vi "nanocal -- nuclear schottky fit V4.vi"() -> ()   [LabVIEW 2020] (continued)
\"mm2\"-> 0.000000000000  , \"mm3\"-> 0.000000000000  , \"T\"->  1.130000000000  , \"B\"-> 12.000000000000  , \"θ\"-> 60.000000000000  |>   , \r\"IDS0371_210908_RAW_cal__ref_\" ->   <| \"ζ\"->  0.020664849580  , \"τ1\"-> 0.018108723176  , \"τS\"-> 0.010299896170  , \"τN\"-> 0.000079818017  , \"τC\"-> 0.006259144045  , \"κ0\"-> 0.000000013130  , \"mm1\"-> 0.000000000000  , \"mm2\"-> 0.000000000000  , \"mm3\"-> 0.000000000000  , \"T\"->  1.900000000000  , \"B\"-> 12.000000000000  , \"θ\"-> 60.000000000000  |>   , \r\"IDS0371_210908_RAW_cal__sam_\" ->   <| \"ζ\"->  0.000000000000  , \"τ1\"-> 0.000000000000  , \"τS\"-> 0.000000000000  , \"τN\"-> 0.000000000000  , \"τC\"-> 0.000000000000  , \"κ0\"-> 0.000000000000  , \"mm1\"-> 0.000000000000  , \"mm2\"-> 0.000000000000  , \"mm3\"-> 0.000000000000  , \"T\"->  1.900000000000  , \"B\"-> 12.000000000000  , \"θ\"-> 60.000000000000  |>   , \r\"IDS0372_210908_RAW_cal__ref_\" ->   <| \"ζ\"->  0.021592146431  , \"τ1\"-> 0.018093446545  , \"τS\"-> 0.007071841556  , \"τN\"-> 0.000029085223  , \"τC\"-> 0.005341206531  , \"κ0\"-> 0.000000023517  , \"mm1\"-> 0.000000000000  , \"mm2\"-> 0.000000000000  , \"mm3\"-> 0.000000000000  , \"T\"->  3.110000000000  , \"B\"-> 12.000000000000  , \"θ\"-> 60.000000000000  |>   , \r\"IDS0372_210908_RAW_cal__sam_\" ->   <| \"ζ\"->  0.000000000000  , \"τ1\"-> 0.000000000000  , \"τS\"-> 0.000000000000  , \"τN\"-> 0.000000000000  , \"τC\"-> 0.000000000000  , \"κ0\"-> 0.000000000000  , \"mm1\"-> 0.000000000000  , \"mm2\"-> 0.000000000000  , \"mm3\"-> 0.000000000000  , \"T\"->  3.110000000000  , \"B\"-> 12.000000000000  , \"θ\"-> 60.000000000000  |>   , \r\"IDS0373_210908_RAW_cal__ref_\" ->   <| \"ζ\"->  0.028148688120  , \"τ1\"-> 0.012706961955  , \"τS\"-> 0.003881518121  , \"τN\"-> 0.000007160132  , \"τC\"-> 0.004346615253  , \"κ0\"-> 0.000000058313  , \"mm1\"-> 0.000000000000  , \"mm2\"-> 0.000000000000  , \"mm3\"-> 0.000000000000  , \"T\"->  5.750000000000  , \"B\"-> 12.000000000000  , \"θ\"-> 60.000000000000  |>   , \r\"IDS0373_210908_RAW_cal__sam_\" ->   <| \"ζ\"->  0.000000000000  , \"τ1\"-> 0.000000000000  , \"τS\"-> 0.000000000000  , \"τN\"-> 0.000000000000  , \"τC\"-> 0.000000000000  , \"κ0\"-> 0.000000000000  , \"mm1\"-> 0.000000000000  , \"mm2\"-> 0.000000000000  , \"mm3\"-> 0.000000000000  , \"T\"->  5.750000000000  , \"B\"-> 12.000000000000  , \"θ\"-> 60.000000000000  |>   , \r\"IDS0377_210909_RAW_cal__ref_\" ->   <| \"ζ\"->  0.217996441376  , \"τ1\"-> 0.079837328848  , \"τS\"-> 0.035140385542  , \"τN\"-> 0.027062270101  , \"τC\"-> 0.001091238478  , \"κ0\"-> 0.000000001044  , \"mm1\"-> 0.000000000000  , \"mm2\"-> 0.000000000000  , \"mm3\"-> 0.000000000000  , \"T\"->  0.197000000000  , \"B\"-> 8.000000000000  , \"θ\"-> 0.000000000000  |>   , \r\"IDS0377_210909_RAW_cal__sam_\" ->   <| \"ζ\"->  0.132375437908  , \"τ1\"-> 0.085614291193  , \"τS\"-> 0.046888304266  , \"τN\"-> 0.035744833495  , \"τC\"-> 0.001504622490  , \"κ0\"-> 0.000000001156  , \"mm1\"-> 0.000000000000  , \"mm2\"-> 0.000000000000  , \"mm3\"-> 0.000000000000  , \"T\"->  0.197000000000  , \"B\"-> 8.000000000000  , \"θ\"-> 0.000000000000  |>   , \r\"IDS0378_210909_RAW_cal__ref_\" ->   <| \"ζ\"->  0.444097524539  , \"τ1\"-> 0.128858676931  , \"τS\"-> 0.109017650637  , \"τN\"-> 0.152310736136  , \"τC\"-> 0.001225116605  , \"κ0\"-> 0.000000000395  , \"mm1\"-> 0.000000000000  , \"mm2\"-> 0.000000000000  , \"mm3\"-> 0.000000000000  , \"T\"->  0.122000000000  , \"B\"-> 8.000000000000  , \"θ\"-> 0.000000000000  |>   , \r\"IDS0378_210909_RAW_cal__sam_\" ->   <| \"ζ\"->  0.278068103221  , \"τ1\"-> 0.118058810167  , \"τS\"-> 0.149294349958  , \"τN\"-> 0.128211590058  , \"τC\"-> 0.001553934408  , \"κ0\"-> 0.000000000522  , \"mm1\"-> 0.000000000000  , \"mm2\"-> 0.000000000000  , \"mm3\"-> 0.000000000000  , \"T\"->  0.122000000000  , \"B\"-> 8.000000000000  , \"θ\"-> 0.000000000000  |>   , \r\"IDS0379_210909_RAW_cal__ref_\" ->   <| \"ζ\"->  0.358674724692  , \"τ1\"-> 0.106557394659  , \"τS\"-> 0.062757387956  , \"τN\"-> 0.083491977845  , \"τC\"-> 0.001111110425  , \"κ0\"-> 0.000000000629  , \"mm1\"-> 0.000000000000  , \"mm2\"-> 0.000000000000  , \"mm3\"-> 0.000000000000  , \"T\"->  0.148000000000  , \"B\"-> 8.000000000000  , \"θ\"-> 0.000000000000  |>   , \r\"IDS0379_210909_RAW_cal__sam_\" ->   <| \"ζ\"->  0.225754480330  , \"τ1\"-> 0.098523892400  , \"τS\"-> 0.080528394696  , \"τN\"-> 0.096491011881  , \"τC\"-> 0.001394999535  , \"κ0\"-> 0.000000000751  , \"mm1\"-> 0.000000000000  , \"mm2\"-> 0.000000000000  , \"mm3\"-> 0.000000000000  , \"T\"->  0.148000000000  , \"B\"-> 8.000000000000  , \"θ\"-> 0.000000000000  |>   , \r\"IDS0380_210909_RAW_cal__ref_\" ->   <| \"ζ\"->  0.289033994940  , \"τ1\"-> 0.085284172773  , \"τS\"-> 0.050519531224  , \"τN\"-> 0.055850802998  , \"τC\"-> 0.001015487958  , \"κ0\"-> 0.000000000740  , \"mm1\"-> 0.000000000000  , \"mm2\"-> 0.000000000000  , \"mm3\"-> 0.000000000000  , \"T\"->  0.168000000000  , \"B\"-> 8.000000000000  , \"θ\"-> 0.000000000000  |>   , \r\"IDS0380_210909_RAW_cal__sam_\" ->   <| \"ζ\"->  0.175421092430  , \"τ1\"-> 0.089198304544  , \"τS\"-> 0.059713999657  , \"τN\"-> 0.066015553792  , \"τC\"-> 0.001291009219  , \"κ0\"-> 0.000000000858  , \"mm1\"-> 0.000000000000  , \"mm2\"-> 0.000000000000  , \"mm3\"-> 0.000000000000  , \"T\"->  0.168000000000  , \"B\"-> 8.000000000000  , \"θ\"-> 0.000000000000  |>   , \r\"IDS0381_210909_RAW_cal__ref_\" ->   <| \"ζ\"->  0.126932147164  , \"τ1\"-> 0.058068643235  , \"τS\"-> 0.026925290066  , \"τN\"-> 0.010981117446  , \"τC\"-> 0.001219952265  , \"κ0\"-> 0.000000001350  , \"mm1\"-> 0.000000000000  , \"mm2\"-> 0.000000000000  , \"mm3\"-> 0.000000000000  , \"T\"->  0.250000000000  , \"B\"-> 8.000000000000  , \"θ\"-> 0.000000000000  |>   , \r\"IDS0381_210909_RAW_cal__sam_\" ->   <| \"ζ\"->  0.078113399712  , \"τ1\"-> 0.055920008457  , \"τS\"-> 0.035460304856  , \"τN\"-> 0.012612271055  , \"τC\"-> 0.001663430483  , \"κ0\"-> 0.000000001497  , \"mm1\"-> 0.000000000000  , \"mm2\"-> 0.000000000000  , \"mm3\"-> 0.000000000000  , \"T\"->  0.250000000000  , \"B\"-> 8.000000000000  , \"θ\"-> 0.000000000000  |>   , \r\"IDS0382_210909_RAW_cal__ref_\" ->   <| \"ζ\"->  0.087249653273  , \"τ1\"-> 0.047168507247  , \"τS\"-> 0.024336865487  , \"τN\"-> 0.005605961335  , \"τC\"-> 0.001526895316  , \"κ0\"-> 0.000000001730  , \"mm1\"-> 0.000000000000  , \"mm2\"-> 0.000000000000  , \"mm3\"-> 0.000000000000  , \"T\"->  0.300000000000  , \"B\"-> 8.000000000000  , \"θ\"-> 0.000000000000  |>   , \r\"IDS0382_210909_RAW_cal__sam_\" ->   <| \"ζ\"->  0.054029770351  , \"τ1\"-> 0.051440847518  , \"τS\"-> 0.032079834642  , \"τN\"-> 0.007150632998  , \"τC\"-> 0.002202148776  , \"κ0\"-> 0.000000001884  , \"mm1\"-> 0.000000000000  , \"mm2\"-> 0.000000000000  , \"mm3\"-> 0.000000000000  , \"T\"->  0.300000000000  , \"B\"-> 8.000000000000  , \"θ\"-> 0.000000000000  |>   , \r\"IDS0383_210910_RAW_cal__ref_\" ->   <| \"ζ\"->  0.062586766538  , \"τ1\"-> 0.048322657274  , \"τS\"-> 0.023582446152  , \"τN\"-> 0.003596780616  , \"τC\"-> 0.001965770478  , \"κ0\"-> 0.000000002106  , \"mm1\"-> 0.000000000000  , \"mm2\"-> 0.000000000000  , \"mm3\"-> 0.000000000000  , \"T\"->  0.360000000000  , \"B\"-> 8.000000000000  , \"θ\"-> 0.000000000000  |>   , \r\"IDS0383_210910_RAW_cal__sam_\" ->   <| \"ζ\"->  0.038341835326  , \"τ1\"-> 0.050866858713  , \"τS\"-> 0.030652081909  , \"τN\"-> 0.004623805952  , \"τC\"-> 0.002823684758  , \"κ0\"-> 0.000000002289  , \"mm1\"-> 0.000000000000  , \"mm2\"-> 0.000000000000  , \"mm3\"-> 0.000000000000  , \"T\"->  0.360000000000  , \"B\"-> 8.000000000000  , \"θ\"-> 0.000000000000  |>   , \r\"IDS0384_210910_RAW_cal__ref_\" ->   <| \"ζ\"->  0.047320664202  , \"τ1\"-> 0.050730770684  , \"τS\"-> 0.023716512211  , \"τN\"-> 0.002200072160  , \"τC\"-> 0.002249629457  , \"κ0\"-> 0.000000002636  , \"mm1\"-> 0.000000000000  , \"mm2\"-> 0.000000000000  , \"mm3\"-> 0.000000000000  , \"T\"->  0.430000000000  , \"B\"-> 8.000000000000  , \"θ\"-> 0.000000000000  |>   , \r\"IDS0384_210910_RAW_cal__sam_\" ->   <| \"ζ\"->  0.029950572027  , \"τ1\"-> 0.044923259835  , \"τS\"-> 0.030416367718  , \"τN\"-> 0.002541256331  , \"τC\"-> 0.003331031560  , \"κ0\"-> 0.000000002858  , \"mm1\"-> 0.000000000000  , \"mm2\"-> 0.000000000000  , \"mm3\"-> 0.000000000000  , \"T\"->  0.430000000000  , \"B\"-> 8.000000000000  , \"θ\"-> 0.000000000000  |>   , \r\"IDS0385_210910_RAW_cal__ref_\" ->   <| \"ζ\"->  0.037147896010  , \"τ1\"-> 0.047226564206  , \"τS\"-> 0.024619467421  , \"τN\"-> 0.001310789285  , \"τC\"-> 0.002565709752  , \"κ0\"-> 0.000000003275  , \"mm1\"-> 0.000000000000  , \"mm2\"-> 0.000000000000  , \"mm3\"-> 0.000000000000  , \"T\"->  0.530000000000  , \"B\"-> 8.000000000000  , \"θ\"-> 0.000000000000  |>   , \r\"IDS0385_210910_RAW_cal__sam_\" ->   <| \"ζ\"->  0.024600756648  , \"τ1\"-> 0.043958236582  , \"τS\"-> 0.031312750224  , \"τN\"-> 0.001348105931  , \"τC\"-> 0.003635120795  , \"κ0\"-> 0.000000003548  , \"mm1\"-> 0.000000000000  , \"mm2\"-> 0.000000000000  , \"mm3\"-> 0.000000000000  , \"T\"->  0.530000000000  , \"B\"-> 8.000000000000  , \"θ\"-> 0.000000000000  |>   , \r\"IDS0386_210910_RAW_cal__ref_\" ->   <| \"ζ\"->  0.028995432115  , \"τ1\"-> 0.046559455187  , \"τS\"-> 0.026126949833  , \"τN\"-> 0.000676599034  , \"τC\"-> 0.003300199116  , \"κ0\"-> 0.000000003897  , \"mm1\"-> 0.000000000000  , \"mm2\"-> 0.000000000000  , \"mm3\"-> 0.000000000000  , \"T\"->  0.630000000000  , \"B\"-> 8.000000000000  , \"θ\"-> 0.000000000000  |>   , \r\"IDS0386_210910_RAW_cal__sam_\" ->   <| \"ζ\"->  0.019494767421  , \"τ1\"-> 0.040349410363  , \"τS\"-> 0.033202805363  , \"τN\"-> 0.000770756985  , \"τC\"-> 0.004303152006  , \"κ0\"-> 0.000000004241  , \"mm1\"-> 0.000000000000  , \"mm2\"-> 0.000000000000  , \"mm3\"-> 0.000000000000  , \"T\"->  0.630000000000  , \"B\"-> 8.000000000000  , \"θ\"-> 0.000000000000  |>   , \r\"IDS0387_210910_RAW_cal__ref_\" ->   <| \"ζ\"->  0.021158107821  , \"τ1\"-> 0.047181877660  , \"τS\"-> 0.030519366684  , \"τN\"-> 0.000257878410  , \"τC\"-> 0.004211881541  , \"κ0\"-> 0.000000005418  , \"mm1\"-> 0.000000000000  , \"mm2\"-> 0.000000000000  , \"mm3\"-> 0.000000000000  , \"T\"->  0.830000000000  , \"B\"-> 8.000000000000  , \"θ\"-> 0.000000000000  |>   , \r\"IDS0387_210910_RAW_cal__sam_\" ->   <| \"ζ\"->  0.013958531253  , \"τ1\"-> 0.040449551738  , \"τS\"-> 0.038075316972  , \"τN\"-> 0.000218997482  , \"τC\"-> 0.005348147372  , \"κ0\"-> 0.000000005866  , \"mm1\"-> 0.000000000000  , \"mm2\"-> 0.000000000000  , \"mm3\"-> 0.000000000000  , \"T\"->  0.830000000000  , \"B\"-> 8.000000000000  , \"θ\"-> 0.000000000000  |>   , \r\"IDS0388_210910_RAW_cal__ref_\" ->   <| \"ζ\"->  0.017074092265  , \"τ1\"-> 0.047215899415  , \"τS\"-> 0.039490388664  , \"τN\"-> 0.000122819272  , \"τC\"-> 0.004722965607  , \"κ0\"-> 0.000000007547  , \"mm1\"-> 0.000000000000  , \"mm2\"-> 0.000000000000  , \"mm3\"-> 0.000000000000  , \"T\"->  1.130000000000  , \"B\"-> 8.000000000000  , \"θ\"-> 0.000000000000  |>   , \r\"IDS0388_210910_RAW_cal__sam_\" ->   <| \"ζ\"->  0.011551866824  , \"τ1\"-> 0.040411227639  , \"τS\"-> 0.048181354691  , \"τN\"-> 0.000103559724  , \"τC\"-> 0.006232382617  , \"κ0\"-> 0.000000008161  , \"mm1\"-> 0.000000000000  , \"mm2\"-> 0.000000000000  , \"mm3\"-> 0.000000000000  , \"T\"->  1.130000000000  , \"B\"-> 8.000000000000  , \"θ\"-> 0.000000000000  |>   , \r\"IDS0389_210910_RAW_cal__ref_\" ->   <| \"ζ\"->  0.017157539727  , \"τ1\"-> 0.046379456311  , \"τS\"-> 0.015264158508  , \"τN\"-> 0.000057006071  , \"τC\"-> 0.004702188691  , \"κ0\"-> 0.000000010470  , \"mm1\"-> 0.000000000000  , \"mm2\"-> 0.000000000000  , \"mm3\"-> 0.000000000000  , \"T\"->  1.520000000000  , \"B\"-> 8.000000000000  , \"θ\"-> 0.000000000000  |>   , \r\"IDS0389_210910_RAW_cal__sam_\" ->   <| \"ζ\"->  0.011148198813  , \"τ1\"-> 0.038849151842  , \"τS\"-> 0.019213865355  , \"τN\"-> 0.000045035153  , \"τC\"-> 0.005536708133  , \"κ0\"-> 0.000000011229  , \"mm1\"-> 0.000000000000  , \"mm2\"-> 0.000000000000  , \"mm3\"-> 0.000000000000  , \"T\"->  1.520000000000  , \"B\"-> 8.000000000000  , \"θ\"-> 0.000000000000  |>   , \r\"IDS0390_210910_RAW_cal__ref_\" ->   <| \"ζ\"->  0.016425367394  , \"τ1\"-> 0.039829137916  , \"τS\"-> 0.010121167967  , \"τN\"-> 0.000033814494  , \"τC\"-> 0.004533563026  , \"κ0\"-> 0.000000013089  , \"mm1\"-> 0.000000000000  , \"mm2\"-> 0.000000000000  , \"mm3\"-> 0.000000000000  , \"T\"->  1.900000000000  , \"B\"-> 8.000000000000  , \"θ\"-> 0.000000000000  |>   , \r\"IDS0390_210910_RAW_cal__sam_\" ->   <| \"ζ\"->  0.010826949430  , \"τ1\"-> 0.038768037521  , \"τS\"-> 0.012925317198  , \"τN\"-> 0.000029157336  , \"τC\"-> 0.005196063884  , \"κ0\"-> 0.000000013864  , \"mm1\"-> 0.000000000000  , \"mm2\"-> 0.000000000000  , \"mm3\"-> 0.000000000000  , \"T\"->  1.900000000000  , \"B\"-> 8.000000000000  , \"θ\"-> 0.000000000000  |>   , \r\"IDS0391_210910_RAW_cal__ref_\" ->   <| \"ζ\"->  0.016160769926  , \"τ1\"-> 0.047360928893  , \"τS\"-> 0.041725389227  , \"τN\"-> 0.000076715950  , \"τC\"-> 0.004871049589  , \"κ0\"-> 0.000000008346  , \"mm1\"-> 0.000000000000  , \"mm2\"-> 0.000000000000  , \"mm3\"-> 0.000000000000  , \"T\"->  1.250000000000  , \"B\"-> 8.000000000000  , \"θ\"-> 0.000000000000  |>   , \r\"IDS0391_210910_RAW_cal__sam_\" ->   <| \"ζ\"->  0.010962610928  , \"τ1\"-> 0.040398807374  , \"τS\"-> 0.051328988590  , \"τN\"-> 0.000070281011  , \"τC\"-> 0.006422533164  , \"κ0\"-> 0.000000008958  , \"mm1\"-> 0.000000000000  , \"mm2\"-> 0.000000000000  , \"mm3\"-> 0.000000000000  , \"T\"->  1.250000000000  , \"B\"-> 8.000000000000  , \"θ\"-> 0.000000000000  |>   , \r\"IDS0392_210910_RAW_cal__ref_\" ->   <| \"ζ\"->  0.016250541117  , \"τ1\"-> 0.047393343666  , \"τS\"-> 0.029998719281  , \"τN\"-> 0.000076850447  , \"τC\"-> 0.004810494325  , \"κ0\"-> 0.000000009475  , \"mm1\"-> 0.000000000000  , \"mm2\"-> 0.000000000000  , \"mm3\"-> 0.000000000000  , \"T\"->  1.390000000000  , \"B\"-> 8.000000000000  , \"θ\"-> 0.000000000000  |>   , \r\"IDS0392_210910_RAW_cal__sam_\" ->   <| \"ζ\"->  0.010962610928  , \"τ1\"-> 0.040398807374  , \"τS\"-> 0.051328988590  , \"τN\"-> 0.000070281011  , \"τC\"-> 0.006422533164  , \"κ0\"-> 0.000000008958  , \"mm1\"-> 0.000000000000  , \"mm2\"-> 0.000000000000  , \"mm3\"-> 0.000000000000  , \"T\"->  1.390000000000  , \"B\"-> 8.000000000000  , \"θ\"-> 0.000000000000  |>   , \r\"IDS0393_210910_RAW_cal__ref_\" ->   <| \"ζ\"->  0.015227705493  , \"τ1\"-> 0.038797003927  , \"τS\"-> 0.007286355621  , \"τN\"-> 0.000013994204  , \"τC\"-> 0.003959851165  , \"κ0\"-> 0.000000023455  , \"mm1\"-> 0.000000000000  , \"mm2\"-> 0.000000000000  , \"mm3\"-> 0.000000000000  , \"T\"->  3.110000000000  , \"B\"-> 8.000000000000  , \"θ\"-> 0.000000000000  |>   , \r\"IDS0393_210910_RAW_cal__sam_\" ->   <| \"ζ\"->  0.010962610928  , \"τ1\"-> 0.040398807374  , \"τS\"-> 0.051328988590  , \"τN\"-> 0.000070281011  , \"τC\"-> 0.006422533164  , \"κ0\"-> 0.000000008958  , \"mm1\"-> 0.000000000000  , \"mm2\"-> 0.000000000000  , \"mm3\"-> 0.000000000000  , \"T\"->  3.110000000000  , \"B\"-> 8.000000000000  , \"θ\"-> 0.000000000000  |>   , \r\"IDS0394_210910_RAW_cal__ref_\" ->   <| \"ζ\"->  0.018884017265  , \"τ1\"-> 0.038756536887  , \"τS\"-> 0.005123025136  , \"τN\"-> 0.000004793994  , \"τC\"-> 0.002621800478  , \"κ0\"-> 0.000000058143  , \"mm1\"-> 0.000000000000  , \"mm2\"-> 0.000000000000  , \"mm3\"-> 0.000000000000  , \"T\"->  5.750000000000  , \"B\"-> 8.000000000000  , \"θ\"-> 0.000000000000  |>   , \r\"IDS0394_210910_RAW_cal__sam_\" ->   <| \"ζ\"->  0.010962610928  , \"τ1\"-> 0.040398807374  , \"τS\"-> 0.051328988590  , \"τN\"-> 0.000070281011  , \"τC\"-> 0.006422533164  , \"κ0\"-> 0.000000008958  , \"mm1\"-> 0.000000000000  , \"mm2\"-> 0.000000000000  , \"mm3\"-> 0.000000000000  , \"T\"->  5.750000000000  , \"B\"-> 8.000000000000  , \"θ\"-> 0.000000000000  |>   , \r\"IDS0395_210910_RAW_cal__ref_\" ->   <| \"ζ\"->  0.016101273075  , \"τ1\"-> 0.047373144247  , \"τS\"-> 0.040453117489  , \"τN\"-> 0.000076678480  , \"τC\"-> 0.005036745304  , \"κ0\"-> 0.000000008627  , \"mm1\"-> 0.000000000000  , \"mm2\"-> 0.000000000000  , \"mm3\"-> 0.000000000000  , \"T\"->  1.310000000000  , \"B\"-> 8.000000000000  , \"θ\"-> 0.000000000000  |>   , \r\"IDS0395_210910_RAW_cal__sam_\" ->   <| \"ζ\"->  0.010962610928  , \"τ1\"-> 0.040398807374  , \"τS\"-> 0.051328988590  , \"τN\"-> 0.000070281011  , \"τC\"-> 0.006422533164  , \"κ0\"-> 0.000000008958  , \"mm1\"-> 0.000000000000  , \"mm2\"-> 0.000000000000  , \"mm3\"-> 0.000000000000  , \"T\"->  1.310000000000  , \"B\"-> 8.000000000000  , \"θ\"-> 0.000000000000  |>   , \r"
  in  "Math --> string OUT  ! :s":bool
  in  "string IN  --> Math!":bool
  in  "file pattern":string="IDS*RAW*_raw_.dat"
  in  "folder":path=path "/opt/new/Dropbox/shared_AkashAndreas/paper-CeCoIn5/Original RAW data"
  in  "filenames":u16(ring)=29 caption="files" items=["IDS0183_210310_RAW_cal_CeCoIn5_2nd_071_12T_0.120K_90deg_Tdep_raw_.dat", "IDS0311_210901_RAW_cal_CeCoIn5_4th_040(126)_C(f)_12T_0.120K_45deg_Tdep_raw_.dat", "IDS0359_210907_RAW_cal_CeCoIn5_4th_089_C(f)_12.0T_0.12K_60deg_Tdep_raw_.dat", "IDS0336_210904_RAW_cal_CeCoIn5_4th_065_C(f)_5.0T_0.122K_90deg_fsweep_Tdep_raw_.dat", "IDS0346_210904_RAW_cal_CeCoIn5_4th_075_C(f)_8.0T_0.122K_90deg_Tdep_raw_.dat", "IDS0378_210909_RAW_cal_CeCoIn5_4th_108_C(f)_8.0T_0.122K_0deg_Tdep_raw_.dat", "IDS0158_210310_RAW_cal_CeCoIn5_2nd_047_12T_fsweep_final_0.14K_0deg_Tdep_raw_.dat", "IDS0300_210427_RAW_cal_CeCoIn5_4th_029(113)_C(f)_12T_0.14K_30deg_NEW_Tdep_raw_.dat", "IDS0184_210310_RAW_cal_CeCoIn5_2nd_072_12T_0.148K_90deg_Tdep_raw_.dat", "IDS0210_210310_RAW_cal_CeCoIn5_2nd_098_fsweep_6T_0.148K_Bdep_raw_.dat", "IDS0379_210909_RAW_cal_CeCoIn5_4th_109_C(f)_8.0T_0.148K_0deg_Tdep_raw_.dat", "IDS0360_210907_RAW_cal_CeCoIn5_4th_090_C(f)_12.0T_0.15K_60deg_Tdep_raw_.dat", "IDS0310_210901_RAW_cal_CeCoIn5_4th_039(125)_C(f)_12T_0.157K_45deg_Tdep_raw_.dat", "IDS0337_210904_RAW_cal_CeCoIn5_4th_066_C(f)_5.0T_0.157K_90deg_Tdep_raw_.dat", "IDS0347_210906_RAW_cal_CeCoIn5_4th_076_C(f)_8.0T_0.157K_90deg_Tdep_raw_.dat", "IDS0305_210831_RAW_cal_CeCoIn5_4th_034(110)_C(f)_12T_0.16K_30deg_NEW_Tdep_raw_.dat", "IDS0361_210908_RAW_cal_CeCoIn5_4th_091_C(f)_12.0T_0.168K_60deg_Tdep_raw_.dat", "IDS0380_210909_RAW_cal_CeCoIn5_4th_110_C(f)_8.0T_0.168K_0deg_Tdep_raw_.dat", "IDS0159_210310_RAW_cal_CeCoIn5_2nd_048_12T_fsweep_0.17K_0deg_Tdep_raw_.dat", "IDS0304_210831_RAW_cal_CeCoIn5_4th_033(112)_C(f)_12T_0.17K_30deg_NEW_Tdep_raw_.dat", "IDS0312_210901_RAW_cal_CeCoIn5_4th_041(127)_C(f)_12T_0.170K_45deg_Tdep_raw_.dat", "IDS0338_210904_RAW_cal_CeCoIn5_4th_067_C(f)_5.0T_0.170K_90deg_Tdep_raw_.dat", "IDS0348_210906_RAW_cal_CeCoIn5_4th_077_C(f)_8.0T_0.178K_90deg_Tdep_raw_.dat", "IDS0181_210310_RAW_cal_CeCoIn5_2nd_070_12T_0.179K_90deg_fsweep_Tdep_raw_.dat", "IDS0185_210310_RAW_cal_CeCoIn5_2nd_073_12T_0.197K_90deg_Tdep_raw_.dat", "IDS0208_210310_RAW_cal_CeCoIn5_2nd_096_Hsweep_0.197K_Tdep_raw_.dat", "IDS0209_210310_RAW_cal_CeCoIn5_2nd_097_Hsweep_0.197K_Tdep_raw_.dat", "IDS0211_210310_RAW_cal_CeCoIn5_2nd_099_fsweep_9T_0.197K_Bdep_raw_.dat", "IDS0212_210310_RAW_cal_CeCoIn5_2nd_100_fsweep_11T_0.197K_Bdep_raw_.dat", "IDS0213_210310_RAW_cal_CeCoIn5_2nd_101_fsweep_10T_0.197K_Bdep_raw_.dat", "IDS0214_210310_RAW_cal_CeCoIn5_2nd_102_fsweep_8T_0.197K_Bdep_raw_.dat", "IDS0215_210310_RAW_cal_CeCoIn5_2nd_103_fsweep_7T_0.197K_Bdep_raw_.dat", "IDS0216_210310_RAW_cal_CeCoIn5_2nd_104_fsweep_5T_0.197K_Bdep_raw_.dat", "IDS0217_210310_RAW_cal_CeCoIn5_2nd_105_fsweep_0T_0.197K_Bdep_raw_.dat", "IDS0330_210901_RAW_cal_CeCoIn5_4th_059_C(f)_1T_0.197K_90deg_Bdep_raw_.dat", "IDS0331_210901_RAW_cal_CeCoIn5_4th_060_C(f)_2T_0.197K_90deg_Bdep_raw_.dat", "IDS0335_210904_RAW_cal_CeCoIn5_4th_064_C(f)_5.0T_0.197K_90deg_fsweep_Tdep_raw_.dat", "IDS0362_210908_RAW_cal_CeCoIn5_4th_092_C(f)_12.0T_0.197K_60deg_Tdep_raw_.dat", "IDS0377_210909_RAW_cal_CeCoIn5_4th_107_C(f)_8.0T_0.197K_0deg_Tdep_raw_.dat", "IDS0160_210310_RAW_cal_CeCoIn5_2nd_049_12T_fsweep_0.20K_0deg_Tdep_raw_.dat", "IDS0303_210831_RAW_cal_CeCoIn5_4th_032(114)_C(f)_12T_0.20K_30deg_NEW_Tdep_raw_.dat", "IDS0313_210901_RAW_cal_CeCoIn5_4th_042(128)_C(f)_12T_0.200K_45deg_Tdep_raw_.dat", "IDS0349_210906_RAW_cal_CeCoIn5_4th_078_C(f)_8.0T_0.20K_90deg_Tdep_raw_.dat", "IDS0161_210310_RAW_cal_CeCoIn5_2nd_050_12T_fsweep_0.22K_0deg_Tdep_raw_.dat", "IDS0186_210310_RAW_cal_CeCoIn5_2nd_074_12T_0.249K_90deg_Tdep_raw_.dat", "IDS0302_210831_RAW_cal_CeCoIn5_4th_031(115)_C(f)_12T_0.25K_30deg_NEW_Tdep_raw_.dat", "IDS0363_210908_RAW_cal_CeCoIn5_4th_093_C(f)_12.0T_0.25K_60deg_Tdep_raw_.dat", "IDS0381_210909_RAW_cal_CeCoIn5_4th_111_C(f)_8.0T_0.25K_0deg_Tdep_raw_.dat", "IDS0314_210901_RAW_cal_CeCoIn5_4th_043(129)_C(f)_12T_0.255K_45deg_Tdep_raw_.dat", "IDS0339_210904_RAW_cal_CeCoIn5_4th_068_C(f)_5.0T_0.255K_90deg_Tdep_raw_.dat", "IDS0350_210906_RAW_cal_CeCoIn5_4th_079_C(f)_8.0T_0.26K_90deg_Tdep_raw_.dat", "IDS0162_210310_RAW_cal_CeCoIn5_2nd_051_12T_fsweep_0.28K_0deg_Tdep_raw_.dat", "IDS0187_210310_RAW_cal_CeCoIn5_2nd_075_12T_0.300K_90deg_Tdep_raw_.dat", "IDS0301_210831_RAW_cal_CeCoIn5_4th_030(116)_C(f)_12T_0.30K_30deg_NEW_Tdep_raw_.dat", "IDS0315_210901_RAW_cal_CeCoIn5_4th_044(130)_C(f)_12T_0.300K_45deg_Tdep_raw_.dat", "IDS0382_210909_RAW_cal_CeCoIn5_4th_112_C(f)_8.0T_0.30K_0deg_Tdep_raw_.dat", "IDS0364_210908_RAW_cal_CeCoIn5_4th_094_C(f)_12.0T_0.307K_60deg_Tdep_raw_.dat", "IDS0340_210904_RAW_cal_CeCoIn5_4th_069_C(f)_5.0T_0.308K_90deg_Tdep_raw_.dat", "IDS0351_210906_RAW_cal_CeCoIn5_4th_080_C(f)_8.0T_0.31K_90deg_Tdep_raw_.dat", "IDS0163_210310_RAW_cal_CeCoIn5_2nd_052_12T_fsweep_0.33K_0deg_Tdep_raw_.dat", "IDS0188_210310_RAW_cal_CeCoIn5_2nd_076_12T_0.360K_90deg_Tdep_raw_.dat", "IDS0299_210427_RAW_cal_CeCoIn5_4th_028(117)_C(f)_12T_0.36K_30deg_NEW_Tdep_raw_.dat", "IDS0316_210901_RAW_cal_CeCoIn5_4th_045(131)_C(f)_12T_0.360K_45deg_Tdep_raw_.dat", "IDS0341_210904_RAW_cal_CeCoIn5_4th_070_C(f)_5.0T_0.360K_90deg_Tdep_raw_.dat", "IDS0352_210906_RAW_cal_CeCoIn5_4th_081_C(f)_8.0T_0.36K_90deg_Tdep_raw_.dat", "IDS0365_210908_RAW_cal_CeCoIn5_4th_095_C(f)_12.0T_0.36K_60deg_Tdep_raw_.dat", "IDS0383_210910_RAW_cal_CeCoIn5_4th_113_C(f)_8.0T_0.36K_0deg_Tdep_raw_.dat", "IDS0164_210310_RAW_cal_CeCoIn5_2nd_053_12T_fsweep_0.40K_0deg_Tdep_raw_.dat", "IDS0189_210310_RAW_cal_CeCoIn5_2nd_077_12T_0.430K_90deg_Tdep_raw_.dat", "IDS0298_210427_RAW_cal_CeCoIn5_4th_027(118)_C(f)_12T_0.43K_30deg_NEW_Tdep_raw_.dat", "IDS0317_210901_RAW_cal_CeCoIn5_4th_046(132)_C(f)_12T_0.43K_45deg_Tdep_raw_.dat", "IDS0366_210908_RAW_cal_CeCoIn5_4th_096_C(f)_12.0T_0.43K_60deg_Tdep_raw_.dat", "IDS0384_210910_RAW_cal_CeCoIn5_4th_114_C(f)_8.0T_0.43K_0deg_Tdep_raw_.dat", "IDS0342_210904_RAW_cal_CeCoIn5_4th_071_C(f)_5.0T_0.438K_90deg_Tdep_raw_.dat", "IDS0353_210906_RAW_cal_CeCoIn5_4th_082_C(f)_8.0T_0.438K_90deg_Tdep_raw_.dat", "IDS0165_210310_RAW_cal_CeCoIn5_2nd_054_12T_fsweep_0.48K_0deg_Tdep_raw_.dat", "IDS0190_210310_RAW_cal_CeCoIn5_2nd_078_12T_0.512K_90deg_Tdep_raw_.dat", "IDS0297_210427_RAW_cal_CeCoIn5_4th_026(119)_C(f)_12T_0.53K_30deg_NEW_Tdep_raw_.dat", "IDS0318_210901_RAW_cal_CeCoIn5_4th_047(133)_C(f)_12T_0.53K_45deg_Tdep_raw_.dat", "IDS0343_210904_RAW_cal_CeCoIn5_4th_072_C(f)_5.0T_0.53K_90deg_Tdep_raw_.dat", "IDS0354_210906_RAW_cal_CeCoIn5_4th_083_C(f)_8.0T_0.53K_90deg_Tdep_raw_.dat", "IDS0367_210908_RAW_cal_CeCoIn5_4th_097_C(f)_12.0T_0.53K_60deg_Tdep_raw_.dat", "IDS0385_210910_RAW_cal_CeCoIn5_4th_115_C(f)_8.0T_0.53K_0deg_Tdep_raw_.dat", "IDS0166_210310_RAW_cal_CeCoIn5_2nd_055_12T_fsweep_0.58K_0deg_Tdep_raw_.dat", "IDS0191_210310_RAW_cal_CeCoIn5_2nd_079_12T_0.610K_90deg_Tdep_raw_.dat", "IDS0296_210427_RAW_cal_CeCoIn5_4th_025(120)_C(f)_12T_0.62K_30deg_NEW_Tdep_raw_.dat", "IDS0319_210901_RAW_cal_CeCoIn5_4th_048(134)_C(f)_12T_0.62K_45deg_Tdep_raw_.dat", "IDS0344_210904_RAW_cal_CeCoIn5_4th_073_C(f)_5.0T_0.62K_90deg_Tdep_raw_.dat", "IDS0368_210908_RAW_cal_CeCoIn5_4th_098_C(f)_12.0T_0.63K_60deg_Tdep_raw_.dat", "IDS0386_210910_RAW_cal_CeCoIn5_4th_116_C(f)_8.0T_0.63K_0deg_Tdep_raw_.dat", "IDS0220_210310_RAW_cal_CeCoIn5_2nd_108_fsweep_0T_0.677K_Bdep_raw_.dat", "IDS0167_210310_RAW_cal_CeCoIn5_2nd_056_12T_fsweep_0.68K_0deg_Tdep_raw_.dat", "IDS0192_210310_RAW_cal_CeCoIn5_2nd_080_12T_0.810K_90deg_Tdep_raw_.dat", "IDS0295_210427_RAW_cal_CeCoIn5_4th_024(121)_C(f)_12T_0.83K_30deg_NEW_Tdep_raw_.dat", "IDS0320_210901_RAW_cal_CeCoIn5_4th_049(135)_C(f)_12T_0.83K_45deg_Tdep_raw_.dat", "IDS0355_210906_RAW_cal_CeCoIn5_4th_085_C(f)_8.0T_0.83K_90deg_Tdep_raw_.dat", "IDS0369_210908_RAW_cal_CeCoIn5_4th_099_C(f)_12.0T_0.83K_60deg_Tdep_raw_.dat", "IDS0387_210910_RAW_cal_CeCoIn5_4th_117_C(f)_8.0T_0.83K_0deg_Tdep_raw_.dat", "IDS0168_210310_RAW_cal_CeCoIn5_2nd_057_12T_fsweep_0.91K_0deg_Tdep_raw_.dat", "IDS0219_210310_RAW_cal_CeCoIn5_2nd_107_fsweep_0T_1.0K_Bdep_raw_.dat", "IDS0193_210310_RAW_cal_CeCoIn5_2nd_081_12T_1.1K_90deg_Tdep_raw_.dat", "IDS0294_210427_RAW_cal_CeCoIn5_4th_023(122)_C(f)_12T_1.13K_30deg_NEW_Tdep_raw_.dat", "IDS0321_210901_RAW_cal_CeCoIn5_4th_050(136)_C(f)_12T_1.13K_45deg_Tdep_raw_.dat", "IDS0370_210908_RAW_cal_CeCoIn5_4th_100_C(f)_12.0T_1.13K_60deg_Tdep_raw_.dat", "IDS0388_210910_RAW_cal_CeCoIn5_4th_118_C(f)_8.0T_1.13K_0deg_Tdep_raw_.dat", "IDS0169_210310_RAW_cal_CeCoIn5_2nd_058_12T_fsweep_1.23K_0deg_Tdep_raw_.dat", "IDS0391_210910_RAW_cal_CeCoIn5_4th_121_C(f)_8.0T_1.25K_0deg_Tdep_raw_.dat", "IDS0395_210910_RAW_cal_CeCoIn5_4th_125_C(f)_8.0T_1.31K_0deg_Tdep_raw_.dat", "IDS0392_210910_RAW_cal_CeCoIn5_4th_122_C(f)_8.0T_1.39K_0deg_Tdep_raw_.dat", "IDS0389_210910_RAW_cal_CeCoIn5_4th_119_C(f)_8.0T_1.52K_0deg_Tdep_raw_.dat", "IDS0218_210310_RAW_cal_CeCoIn5_2nd_106_fsweep_0T_1.55K_Bdep_raw_.dat", "IDS0194_210310_RAW_cal_CeCoIn5_2nd_082_12T_1.8K_90deg_Tdep_raw_.dat", "IDS0293_210427_RAW_cal_CeCoIn5_4th_022(123)_C(f)_12T_1.90K_30deg_NEW_Tdep_raw_.dat", "IDS0322_210901_RAW_cal_CeCoIn5_4th_051(137)_C(f)_12T_1.90K_45deg_Tdep_raw_.dat", "IDS0371_210908_RAW_cal_CeCoIn5_4th_101_C(f)_12.0T_1.90K_60deg_Tdep_raw_.dat", "IDS0390_210910_RAW_cal_CeCoIn5_4th_120_C(f)_8.0T_1.90K_0deg_Tdep_raw_.dat", "IDS0170_210310_RAW_cal_CeCoIn5_2nd_059_12T_fsweep_1.97K_0deg_Tdep_raw_.dat", "IDS0195_210310_RAW_cal_CeCoIn5_2nd_083_12T_3.0K_90deg_Tdep_raw_.dat", "IDS0306_210831_RAW_cal_CeCoIn5_4th_035(124)_C(f)_12T_3.10K_30deg_NEW_Tdep_raw_.dat", 
